vi "MultiSerialReaderWriter.vi"() -> ()   [LabVIEW 2015]
uses:
  <vilib>/Instr/_visa.llb/Select Event Type.ctl
  <vilib>/Instr/_visa.llb/VISA Configure Serial Port (Instr).vi
  <vilib>/regexp/Match Regular Expression.xnode
panel:
  out "Serial Feed":string
  out "Last Received":string
  in  "Boolean":bool
  out "Serial Errors":errorcluster {"code" format="%.0x"}
  in  "Start/Stop":bool=TRUE
  in  "VISA resource name":refnum<visa-resource-name>
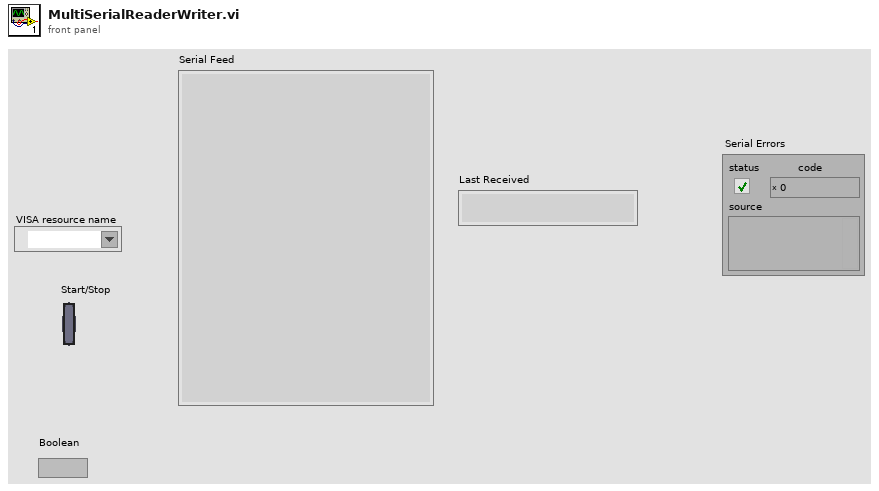
[diagram p1: front panel]
types:
  T1 = typedef "Select Event Type.ctl" = u32
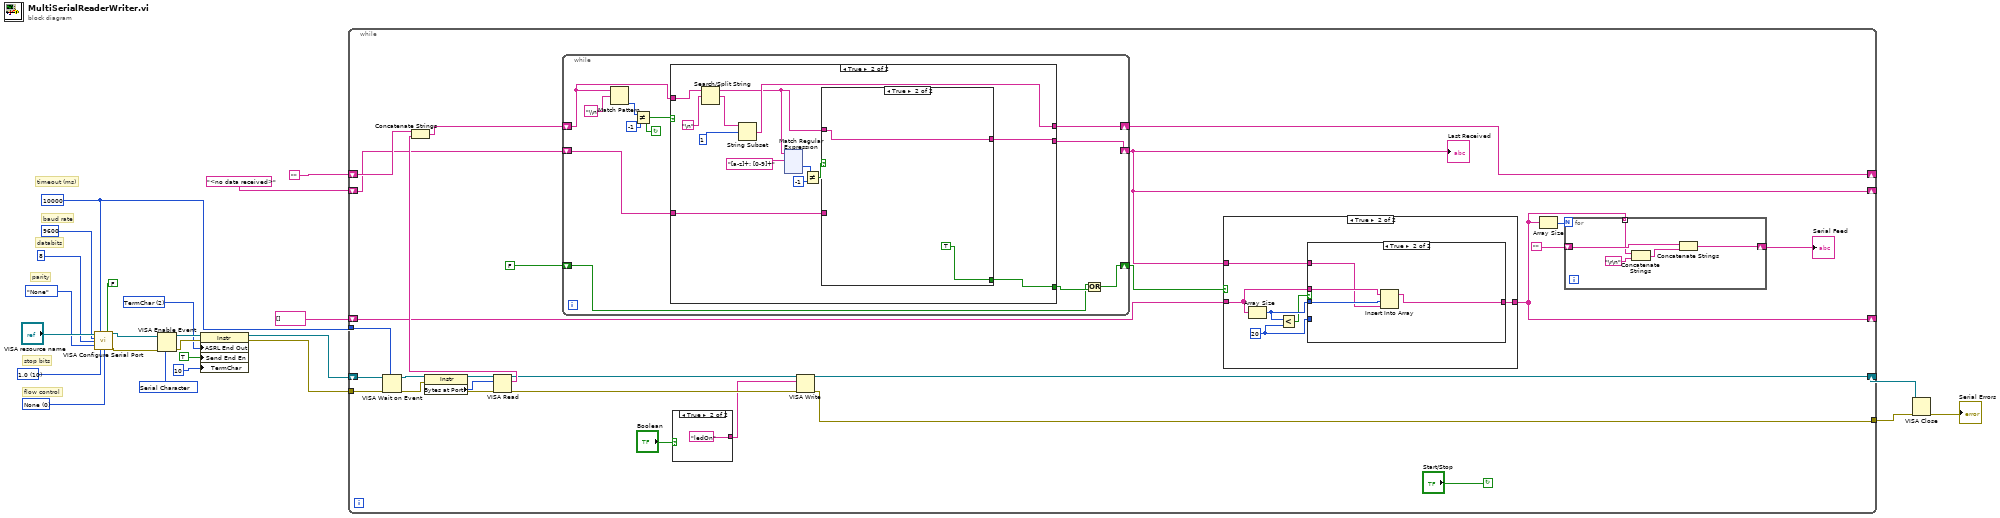
[diagram p0: block diagram]
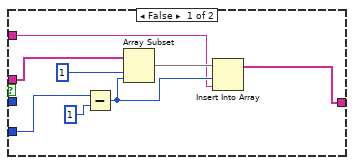
[diagram p3: hidden frame]
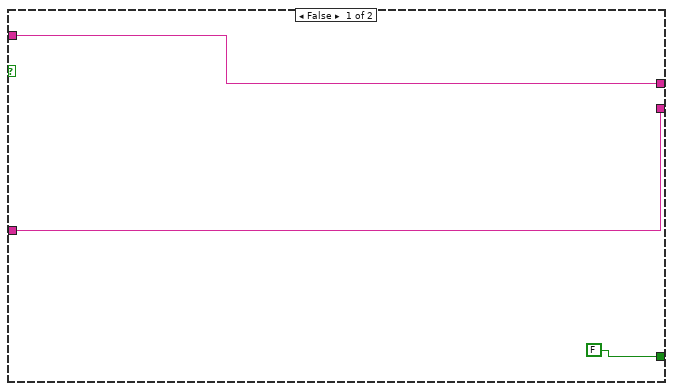
[diagram p4: hidden frame]
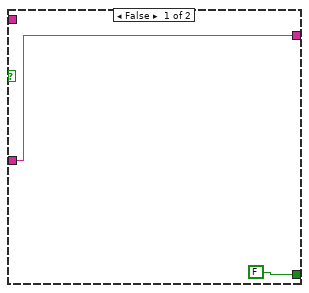
[diagram p5: hidden frame]
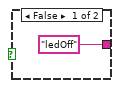
[diagram p6: hidden frame]
diagram:
  w6 = u16 2 items=["None", "LastBit", "TermChar", "Break"] ("Serial Settings:Serial End Mode for Writes")
  w17 = u16 0 items=["None", "XON/XOFF", "RTS/CTS", "XON/XOFF & RTS/CTS", "DTR/DSR", "XON/XOFF & DTR/DSR"] ("flow control (0:none)")
  w18 = u16 10 items=["1.0"=10, "1.5"=15, "2.0"=20] ("stop bits (10: 1 bit)")
  w15 = 10000
  w24 = T1 1073684533 items=["Service Request"=1073684491, "Trigger"=3221168138, "Clear"=1073684493, "VXI Signal"=1073684512, "VXI/VME Interrupt"=3221168161, "VXI/VME Sysfail"=1073684509, "VXI/VME Sysreset"=1073684510, "GPIB CIC"=1073684498, "GPIB Talk"=1073684499, "GPIB Listen"=1073684500, "PXI Interrupt"=1073684514, "Serial Break"=1073684515, "Serial TermChar"=1073684516, "Serial CTS"=1073684521, "Serial DSR"=1073684522, "Serial DCD"=1073684524, "Serial RI"=1073684526, "Serial Character"=1073684533, "USB Interrupt"=1073684535, "All Enabled"=1073709055] ("Event Type")
  # "stop bits"
  # "flow control"
  # "parity"
  # "databits"
  # "baud rate"
  # "timeout (ms)"
  n1 = call-poly "VISA Configure Serial Port"("VISA resource name"="VISA resource name", "timeout (10sec)"=w15, "Enable Termination\nChar (T)"=FALSE ("Enable Termination\nChar (T)"), "baud rate (9600)"=9600, "data bits (8)"=8, "parity (0:none)"=enum16{"None", "Odd", "Even", "Mark", "Space"}."None", "stop bits (10: 1 bit)"=w18, "flow control (0:none)"=w17) -> ("VISA resource name out"=w14:refnum<visa-resource-name>, "error out"=w13:errorcluster)  [unwired: 6 in]
  n2 = VISA Enable Event(8:w13, 10:w24, 11:w14) -> (0:w8:errorcluster, 3:w10:refnum<visa-resource-name>)  [unwired: 1 in]
  n3 = property class="Instr"(reference=w10, error in=w8, "ASRL End Out"=w6, "Send End En"=TRUE, "TermChar"=10) -> (reference out=w9:refnum<visa-resource-name>, error out=w7:errorcluster)
  n4 = while {
    tunnel: w7 -> [w48]
    tunnel: [w38] -> w12
    shift-right: [w34] -> _
    shift-left: "" -> [w50]
    tunnel: w15 -> [w47]
    shift-right: [w37] -> w11
    shift-left: w9 -> [w49]
    shift-right: [w29] -> _
    shift-left: "<no data received>" -> [w33]
    shift-right: [w28] -> _
    shift-left: string[] [] -> [w27]
    stop <- "Start/Stop" continue-if-true
    n5 = VISA Wait on Event(7:w47, 8:w48, 11:w49) -> (0:w45:errorcluster, 3:w46:refnum<visa-resource-name>)  [unwired: 2 in, 2 out]
    n6 = property class="Instr"(reference=w46, error in=w45) -> (reference out=w44:refnum<visa-resource-name>, error out=w43:errorcluster, "Bytes at Port"=w42:u32)
    n7 = VISA Read(VISA resource name=w44, byte count=w42, error in (no error)=w43) -> (VISA resource name out=w40:refnum<visa-resource-name>, read buffer=w51:string, error out=w39:errorcluster)  [unwired: 1 out]
    n8 = Concatenate Strings(w50, w51) -> (w35:string)
    n9 = while {
      shift-right: [w84] -> w34
      shift-left: w35 -> [w82]
      shift-right: [w80] -> w29
      shift-left: w33 -> [w81]
      shift-right: [w77] -> w25
      shift-left: FALSE -> [w78]
      stop <- w85 continue-if-true
      n10 = Match Pattern(string=w82, regular expression="\\n") -> (offset past match=w87:i32)  [unwired: 1 in, 3 out]
      n11 = Not Equal?(x=w87, y=-1) -> (x != y?=w85:bool)
      n12 = case shown="True" w85 {
        tunnel: [w90 w101] -> w84
        tunnel: w82 -> [w90 w100]
        tunnel: w81 -> [w89 w93]
        tunnel: [w89 w92] -> w80
        tunnel: [FALSE w91] -> w79
        frame False {
        }
        frame True {
          n13 = Search/Split String(string=w100, search string/char (-)="\n") -> (substring before match=w94:string, match + rest of string=w103:string)  [unwired: 1 in, 1 out]
          n14 = String Subset(string=w103, offset (0)=1) -> (substring=w101:string)  [unwired: 1 in]
          n15 = xnode "Match Regular Expression"("input string"=w94, "regular expression"="[a-z]+: [0-9]+") -> ("offset past match"=w96:i32)  [unwired: 4 in, 4 out]
          n16 = Not Equal?(x=w96, y=-1) -> (x != y?=w97:bool)
          n17 = case shown="True" w97 {
            tunnel: w94 -> [_ w107]
            tunnel: w93 -> [w105 _]
            tunnel: [w105 w107] -> w92
            tunnel: [FALSE TRUE] -> w91
            frame False {
            }
            frame True {
            }
          }
        }
      }
      n18 = Or(x=w78, y=w79) -> (x .or. y?=w77:bool)
    }
    "Last Received" <- w29
    n19 = case shown="True" "Boolean" {
      tunnel: ["ledOff" "ledOn"] -> w36
      frame False {
      }
      frame True {
      }
    }
    n20 = VISA Write(VISA resource name=w40, write buffer=w36, error in (no error)=w39) -> (VISA resource name out=w37:refnum<visa-resource-name>, error out=w38:errorcluster)  [unwired: 1 out]
    n21 = case shown="True" w25 {
      tunnel: w29 -> [_ w56]
      tunnel: [w53 w55] -> w28
      tunnel: w27 -> [w53 w54]
      frame False {
      }
      frame True {
        w59 = 20
        n22 = Array Size(array=w54) -> (size(s)=w58:i32)
        n23 = Less?(x=w58, y=w59) -> (x < y?=w57:bool)
        n24 = case shown="True" w57 {
          tunnel: w54 -> [w67 w71]
          tunnel: w58 -> [_ w70]
          tunnel: [w61 w69] -> w55
          tunnel: w59 -> [w65 _]
          tunnel: w56 -> [w60 w68]
          frame False {
            n25 = Subtract(x=w65, y=1) -> (x-y=w62:i32)
            n26 = Array Subset(array=w67, index=1, length=w62) -> (w63:string[])
            n27 = Insert Into Array(array=w63, index=w62, new element=w60) -> (w61:string[])
          }
          frame True {
            n28 = Insert Into Array(array=w71, index=w70, new element=w68) -> (w69:string[])
          }
        }
      }
    }
    n29 = Array Size(array=w28) -> (size(s)=w32:i32)
    n30 = for {
      N: w32 -> [_]
      tunnel: w28 -> [w74] mode=indexing
      shift-right: [w75] -> w30
      shift-left: "" -> [w76]
      n31 = Concatenate Strings(w74, "\r\n") -> (w72:string)
      n32 = Concatenate Strings(w76, w72) -> (w75:string)
    }
    "Serial Feed" <- w30
  }
  n33 = VISA Close(VISA resource name=w11, error in (no error)=w12) -> (error out=→"Serial Errors":errorcluster)
